vi "PH_uOPA_DelayController.destructor.vi"(0 "i ref in":refnum<vi>, 5 "error in(no error)":errorcluster) -> (19 "error out":errorcluster)   [LabVIEW 2014, in "PH_uOPA_DelayController.lvlib"]
doc: "This is the destructor of a class.\n\nLicense Agreement for this software:\n\nCopyright (C)\nGesellschaft für Schwerionenforschung, GSI\nPlanckstr. 1\n64291 Darmstadt\nGermany\n\nContact: D.Beck@gsi.de \n\nThis program is free software; you can redistribute it and/or modify it under the terms of the \nGNU General Public License as published by the Free Software Foundation; either version 2 of \nthe license, or (at your option) any later version.\n\nThis program is distributed in the hope that it will be useful, but WITHOUT ANY WARRANTY; \nwithout even the implied warranty of MERCHANTABILITY or FITNESS FOR A PARTICULAR PURPOSE. See the GNU General License for more details (http://www.gnu.org).\n\nGesellschaft für Schwerionenforschung, GSI\nPlanckstr. 1, 64291 Darmstadt, Germany\nFor all questions and ideas contact: M.Richter@gsi.de, H.Brand@gsi.de or D.Beck@gsi.de.\nLast update: 16-JUN-2004"
uses:
  PH_uOPA_DelayController.lvlib
  PH_Devices/PH_TKTDS-30xx/PH_TKTDS-30xx.lvlib
  CS_Core/BaseProcess/BaseProcess.lvlib
  PH_Basics/PH_StatusHandler/PH_StatusHandler.lvlib
  PH_Basics/PH_AxisGUI_BaseClass/PH_AxisGUI_BaseClass.lvlib
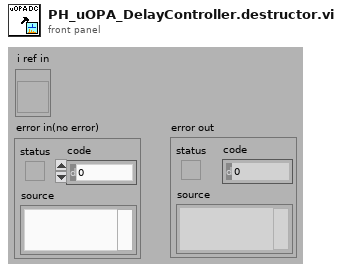
[diagram p1: front panel]
types:
  T1 = typedef "BaseProcess.lvlib/BaseProcess.i attribute.ctl" = cluster{"EventStatus":string, "EventError":i32, "PresetEvtWatchD":i32, "PresetPdcWatchD":i32, "EventTimeout":i32, "PeriodicInterval":i32, "Interface":string[], "Address":string[], "Special":string[], "PeriodicError":i32, "PeriodicStatus":string, "SuperProc":string, "Descriptors":T2[], "CaseRef":refnum<vi>, "PdcRef":refnum<vi>, "Thread Ref":refnum<vi>, "eventErrorID":i32, "eventStatusID":i32, "periodicErrorID":i32, "periodicStatusID":i32, "pdcCtrID":i32}
  T2 = typedef "BaseProcess.lvlib/BaseProcess.descriptor definition.ctl" = cluster{"selector":string, "descriptor":T3}
  T3 = typedef "BaseProcess.lvlib/BaseProcess.descriptor string definition.ctl" = string
  T4 = enum16{"SetAttribute", "GetAttribute", "CreateAttribute", "DestroyAttribute", "DestroyAllAtributes"}
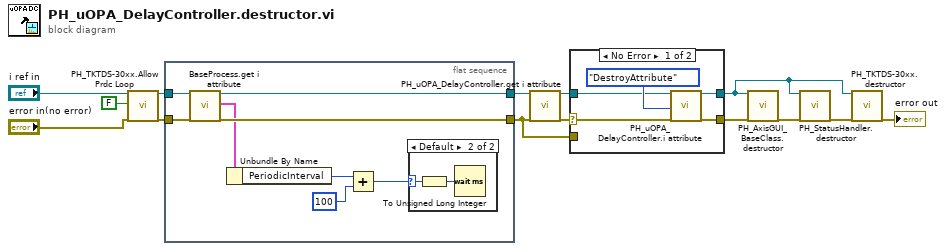
[diagram p0: block diagram]
diagram:
  n1 = call "PH_TKTDS-30xx.Allow Prdc Loop.vi"("i ref in"="i ref in", "Allow Prdc Loop?"=FALSE, "error in"="error in(no error)") -> ("i ref out"=w9:refnum<vi>, "error out"=w8:errorcluster)  [unwired: 15 in]
  n2 = flat-sequence {
    tunnel: w8 -> [w22]
    tunnel: [w21] -> w5
    tunnel: w9 -> [w20]
    tunnel: [w19] -> w7
    frame #0 {
      n3 = call "BaseProcess.get i attribute.vi"("i ref in"=w20, "error in (no error)"=w22) -> ("i ref out"=w19:refnum<vi>, "i attribute"=w18:T1, "error out"=w21:errorcluster)  [unwired: 15 in]
      n4 = Unbundle By Name(w18) -> ("PeriodicInterval"=w17:i32)
      n5 = Add(x=w17, y=100) -> (x+y=w15:i32)
      n6 = case shown="Default" w15 {
        selector: w15 -> [_ w24]
        frame -1 {
        }
        frame Default {
          n7 = To Unsigned Long Integer(number=w24) -> (unsigned 32bit integer=w23:u32)
          n8 = Wait (ms)(milliseconds to wait=w23) -> ()  [unwired: 1 out]
        }
      }
    }
  }
  n9 = call "PH_uOPA_DelayController.get i attribute.vi"("i ref in"=w7, "error in (no error)"=w5) -> ("i ref out"=w12:refnum<vi>, "error out"=w6:errorcluster)  [unwired: 15 in, 1 out]
  n10 = case shown="No Error" w6 {
    selector: w6 -> [w25 _]
    tunnel: [w29 w30] -> w14
    tunnel: w12 -> [w27 w31]
    tunnel: [w26 w31] -> w1
    tunnel: w5 -> [_ w30]
    frame No Error {
      n11 = call "PH_uOPA_DelayController.i attribute.vi"("VI Refnum"=w27, "Action"=T4."DestroyAttribute", "error in (no error)"=w25) -> ("VI Refnum out"=w26:refnum<vi>, "error out"=w29:errorcluster)  [unwired: 14 in, 1 out]
    }
    frame Error {
    }
  }
  n12 = call "PH_AxisGUI_BaseClass.destructor.vi"("i ref in"=w1, "error in(no error)"=w14) -> ("error out"=w2:errorcluster)  [unwired: 17 in]
  n13 = call "PH_StatusHandler.destructor.vi"("i ref in"=w1, "error in(no error)"=w2) -> ("error out"=w3:errorcluster)  [unwired: 17 in]
  n14 = call "PH_TKTDS-30xx.destructor.vi"("i ref in"=w1, "error in(no error)"=w3) -> ("error out"=→"error out":errorcluster)  [unwired: 17 in]
